vi "Frequency Shift.vi"(0 "data in":T1[](array[typedef])=[{"I"=0.0, "Q"=0.0, "overflow"=FALSE}, {"I"=0.0, "Q"=0.0, "overflow"=FALSE}], 9 "input valid":bool, 11 "acq in":refnum<class "niUSRP Rx DSP v2 FPGA.lvclass">, 12 "ready for output (T)":bool=TRUE) -> (4 "data out":T1[](array[typedef]), 10 "output valid":bool, 14 "ready for input":bool, 15 "acq out":refnum<class "niUSRP Rx DSP v2 FPGA.lvclass">)   [LabVIEW 2025, in "niUSRP Rx DSP v2 FPGA.lvclass"]
uses:
  niUSRP Rx DSP v2 FPGA.lvclass
  <instrlib>/_niInstr/DSP/v1/Shared/Public/IQ Data.ctl
  <instrlib>/_niInstr/DSP Control/Interface/v1/FPGA/Frequency Shift/IQ 18-bit/Frequency Shift Interface (IQ 18-bit).lvclass
  <instrlib>/_niInstr/DSP/v1/Shared/niInstr DSP v1 Shared.lvlib
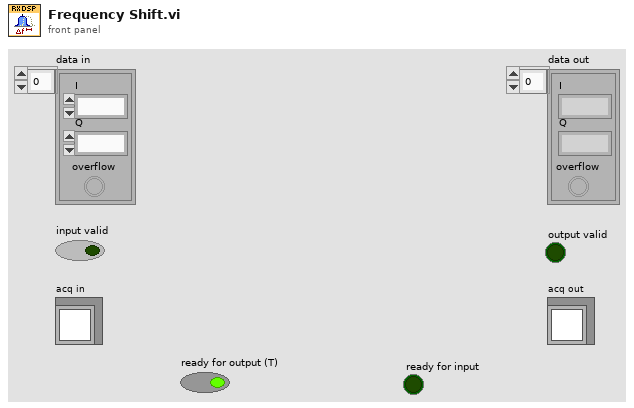
[diagram p1: front panel]
types:
  T1 = typedef "niInstr DSP v1 Shared.lvlib/IQ Data.ctl" = cluster{"I":fxp<+/-,18,1>, "Q":fxp<+/-,18,1>, "overflow":bool}
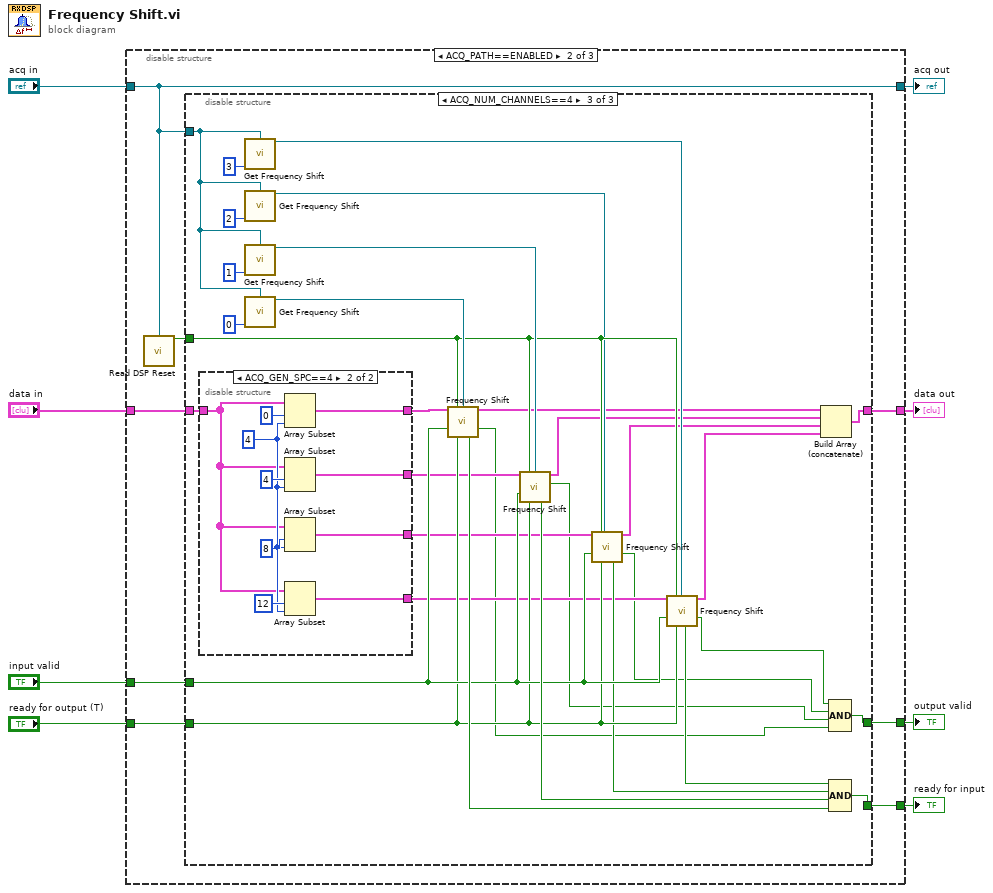
[diagram p0: block diagram]
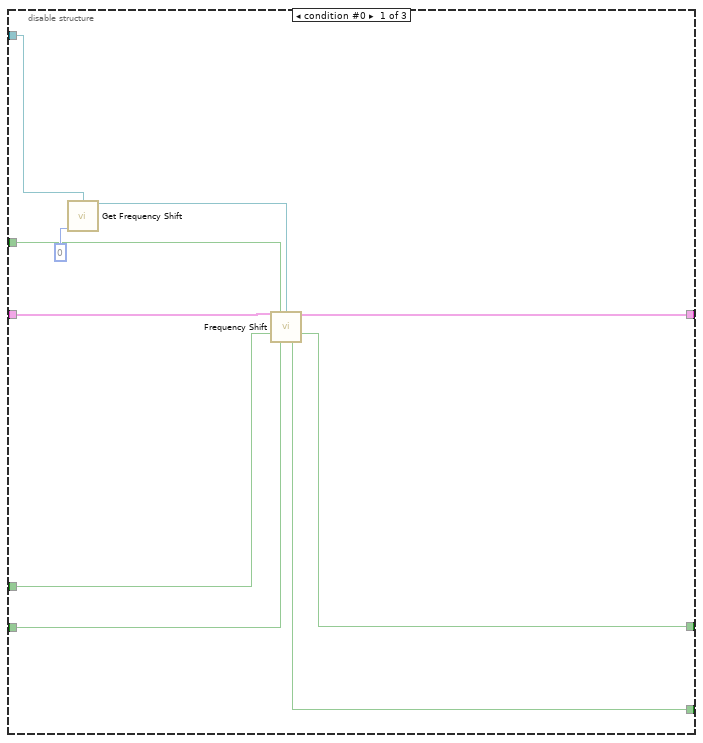
[diagram p3: hidden frame]
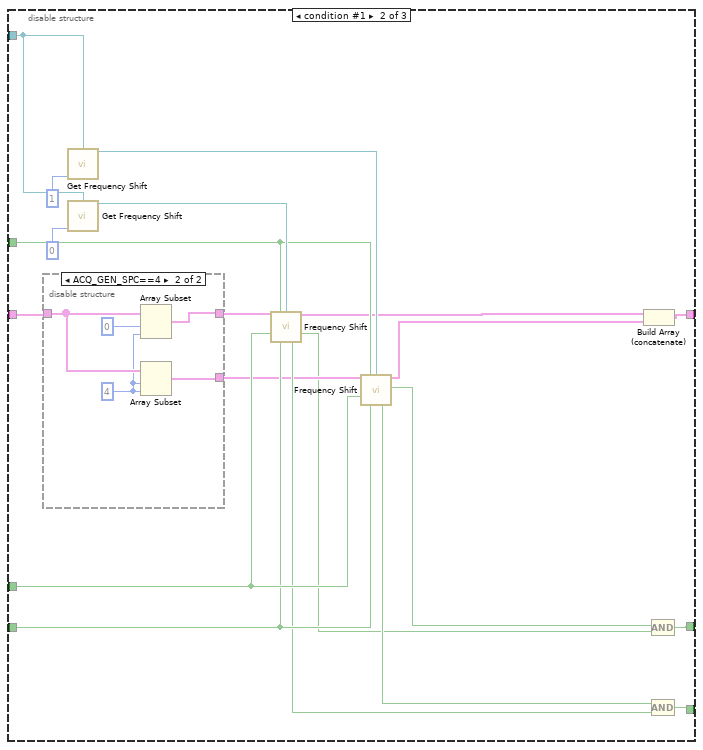
[diagram p4: hidden frame]
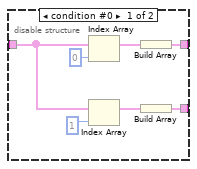
[diagram p5: hidden frame]
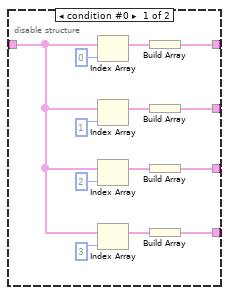
[diagram p6: hidden frame]
diagram:
  n1 = disable-structure shown="ACQ_PATH==ENABLED" {
    disable-tunnel: "data in" -> [_ w10 w116]
    disable-tunnel: [_ w9 w116] -> w7
    disable-tunnel: "input valid" -> [_ w16 w114]
    disable-tunnel: "ready for output (T)" -> [_ w15 w115]
    disable-tunnel: [_ w14 w114] -> w4
    disable-tunnel: "acq in" -> [_ w11 w117]
    disable-tunnel: [_ w11 w117] -> w3
    disable-tunnel: [_ w12 w115] -> w2
    frame condition #0 {
      # "IF YOU REACH THIS STATE:\nlabview has failed to propagate the conditional symbol for this structure. to fix this, edit the condition and click OK (typically, no actual changes are necessary)."
    }
    frame condition #1 (active) {
      n2 = call-dynamic "Read DSP Reset.vi"("acq"=w11) -> ("dsp reset"=w13:bool)  [unwired: 14 in]
      n3 = disable-structure shown="ACQ_NUM_CHANNELS==4" {
        disable-tunnel: w16 -> [w22 w40 w76]
        disable-tunnel: w15 -> [w21 w39 w75]
        disable-tunnel: [w19 w37 w85] -> w14
        disable-tunnel: w13 -> [w23 w41 w79]
        disable-tunnel: [w18 w36 w84] -> w12
        disable-tunnel: w11 -> [w25 w45 w72]
        disable-tunnel: w10 -> [w17 w33 w71]
        disable-tunnel: [w20 w34 w82] -> w9
        frame condition #0 {
          n4 = call-dynamic "Get Frequency Shift.vi"("acq in"=w25, "ch"=u8 0) -> ("frequency shift"=w26:refnum<class "Frequency Shift Interface (IQ 18-bit).lvclass">)  [unwired: 13 in]
          n5 = call-dynamic "Frequency Shift.vi"("data in"=w17, "reset"=w23, "frequency shift"=w26, "input valid"=w22, "ready for output (T)"=w21) -> ("data out"=w20:T1[], "output valid"=w19:bool, "ready for input"=w18:bool)  [unwired: 7 in, 1 out]
        }
        frame condition #1 {
          n6 = disable-structure shown="ACQ_GEN_SPC==4" {
            disable-tunnel: w33 -> [w49 w56]
            disable-tunnel: [w48 w57] -> w32
            disable-tunnel: [w47 w55] -> w31
            frame condition #0 {
              n7 = Index Array(array=w49, index=0) -> (element=w53:T1)
              n8 = Index Array(array=w49, index=1) -> (element=w51:T1)
              n9 = Build Array(w53) -> (w48:T1[])
              n10 = Build Array(w51) -> (w47:T1[])
            }
            frame condition #1 (active) {
              w54 = 4 ("length")
              n11 = Array Subset(array=w56, index=0, length=w54) -> (w57:T1[])
              n12 = Array Subset(array=w56, index=w54, length=w54) -> (w55:T1[])
            }
          }
          n13 = call-dynamic "Get Frequency Shift.vi"("acq in"=w45, "ch"=u8 1) -> ("frequency shift"=w44:refnum<class "Frequency Shift Interface (IQ 18-bit).lvclass">)  [unwired: 13 in]
          n14 = call-dynamic "Get Frequency Shift.vi"("acq in"=w45, "ch"=u8 0) -> ("frequency shift"=w46:refnum<class "Frequency Shift Interface (IQ 18-bit).lvclass">)  [unwired: 13 in]
          n15 = call-dynamic "Frequency Shift.vi"("data in"=w32, "reset"=w41, "frequency shift"=w46, "input valid"=w40, "ready for output (T)"=w39) -> ("data out"=w30:T1[], "output valid"=w27:bool, "ready for input"=w38:bool)  [unwired: 7 in, 1 out]
          n16 = call-dynamic "Frequency Shift.vi"("data in"=w31, "reset"=w41, "frequency shift"=w44, "input valid"=w40, "ready for output (T)"=w39) -> ("data out"=w29:T1[], "output valid"=w28:bool, "ready for input"=w35:bool)  [unwired: 7 in, 1 out]
          n17 = Build Array (concatenate)(w30, w29) -> (w34:T1[])
          n18 = Compound Arithmetic op=AND(w28, w27) -> (w37:bool)
          n19 = Compound Arithmetic op=AND(w35, w38) -> (w36:bool)
        }
        frame condition #2 (active) {
          n20 = disable-structure shown="ACQ_GEN_SPC==4" {
            disable-tunnel: [w99 w107] -> w70
            disable-tunnel: [w98 w106] -> w69
            disable-tunnel: [w97 w105] -> w68
            disable-tunnel: w71 -> [w92 w108]
            disable-tunnel: [w91 w104] -> w67
            frame condition #0 {
              n21 = Index Array(array=w92, index=0) -> (element=w103:T1)
              n22 = Index Array(array=w92, index=1) -> (element=w101:T1)
              n23 = Index Array(array=w92, index=2) -> (element=w93:T1)
              n24 = Index Array(array=w92, index=3) -> (element=w95:T1)
              n25 = Build Array(w103) -> (w99:T1[])
              n26 = Build Array(w101) -> (w98:T1[])
              n27 = Build Array(w93) -> (w97:T1[])
              n28 = Build Array(w95) -> (w91:T1[])
            }
            frame condition #1 (active) {
              w109 = 4 ("length")
              n29 = Array Subset(array=w108, index=0, length=w109) -> (w107:T1[])
              n30 = Array Subset(array=w108, index=4, length=w109) -> (w106:T1[])
              n31 = Array Subset(array=w108, index=8, length=w109) -> (w105:T1[])
              n32 = Array Subset(array=w108, index=12, length=w109) -> (w104:T1[])
            }
          }
          n33 = call-dynamic "Get Frequency Shift.vi"("acq in"=w72, "ch"=u8 3) -> ("frequency shift"=w77:refnum<class "Frequency Shift Interface (IQ 18-bit).lvclass">)  [unwired: 13 in]
          n34 = call-dynamic "Get Frequency Shift.vi"("acq in"=w72, "ch"=u8 2) -> ("frequency shift"=w78:refnum<class "Frequency Shift Interface (IQ 18-bit).lvclass">)  [unwired: 13 in]
          n35 = call-dynamic "Get Frequency Shift.vi"("acq in"=w72, "ch"=u8 1) -> ("frequency shift"=w89:refnum<class "Frequency Shift Interface (IQ 18-bit).lvclass">)  [unwired: 13 in]
          n36 = call-dynamic "Get Frequency Shift.vi"("acq in"=w72, "ch"=u8 0) -> ("frequency shift"=w90:refnum<class "Frequency Shift Interface (IQ 18-bit).lvclass">)  [unwired: 13 in]
          n37 = call-dynamic "Frequency Shift.vi"("data in"=w70, "reset"=w79, "frequency shift"=w90, "input valid"=w76, "ready for output (T)"=w75) -> ("data out"=w66:T1[], "output valid"=w59:bool, "ready for input"=w86:bool)  [unwired: 7 in, 1 out]
          n38 = call-dynamic "Frequency Shift.vi"("data in"=w69, "reset"=w79, "frequency shift"=w89, "input valid"=w76, "ready for output (T)"=w75) -> ("data out"=w65:T1[], "output valid"=w60:bool, "ready for input"=w83:bool)  [unwired: 7 in, 1 out]
          n39 = call-dynamic "Frequency Shift.vi"("data in"=w68, "reset"=w79, "frequency shift"=w78, "input valid"=w76, "ready for output (T)"=w75) -> ("data out"=w64:T1[], "output valid"=w61:bool, "ready for input"=w74:bool)  [unwired: 7 in, 1 out]
          n40 = call-dynamic "Frequency Shift.vi"("data in"=w67, "reset"=w79, "frequency shift"=w77, "input valid"=w76, "ready for output (T)"=w75) -> ("data out"=w63:T1[], "output valid"=w62:bool, "ready for input"=w73:bool)  [unwired: 7 in, 1 out]
          n41 = Build Array (concatenate)(w66, w65, w64, w63) -> (w82:T1[])
          n42 = Compound Arithmetic op=AND(w62, w61, w60, w59) -> (w85:bool)
          n43 = Compound Arithmetic op=AND(w73, w74, w83, w86) -> (w84:bool)
        }
      }
    }
    frame condition #2 {
    }
  }
  "data out" <- w7
  "output valid" <- w4
  "ready for input" <- w2
  "acq out" <- w3
